vi "Coord window-Offset to zero.vi"() -> (0 "error out":errorcluster)   [LabVIEW 2020]
uses:
  Globals/Coord window-Globals.vi
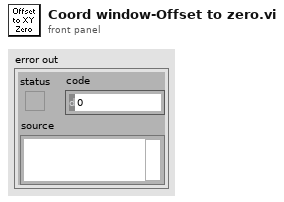
[diagram p1: front panel]
types:
  T1 = typedef "Coordinate list window refs.ctl" = cluster{"Window Name (i.e. Key)":string, "menu reference":refnum<k9>, "VI's reference":refnum<vi>, "Pane 1":refnum<vi>, "Pane 2":refnum<vi>, "Coord Listbox":refnum<vi>, "File name":refnum<vi>, "Picture Map":refnum<vi>, "Stage XYZ Position ind.":refnum<vi>}
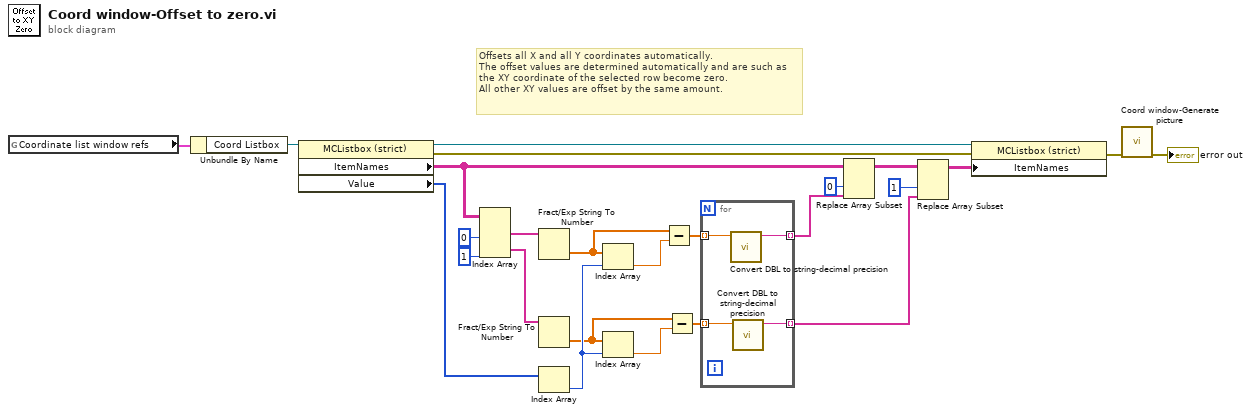
[diagram p0: block diagram]
diagram:
  # "Offsets all X and all Y coordinates automatically.\nThe offset values are determined automatically and are such as the XY coordinate of the selected row become zero.\nAll other XY values are offset by the same amount."
  n1 = global read "Coord window-Globals.vi" "Coordinate list window refs"() -> (w25:T1)
  n2 = Unbundle By Name(w25) -> ("Coord Listbox"=w24:refnum<vi>)
  n3 = property class="MCListbox (strict)"(reference=w24) -> (reference out=w4:refnum<vi>, error out=w3:errorcluster, "ItemNames"=w11:string[][], "Value"=w23:i32[])  [unwired: 1 in]
  n4 = Index Array(array=w11, index (col) #1=0 ("disabled index (col)"), index (col) #2=1 ("index (col)")) -> (element #1=w19:string[], element #2=w18:string[])  [unwired: 2 in]
  n5 = Fract/Exp String To Number(string=w19) -> (number=w17:dbl[])  [unwired: 3 in, 1 out]
  n6 = Fract/Exp String To Number(string=w18) -> (number=w15:dbl[])  [unwired: 3 in, 1 out]
  n7 = Index Array(array=w23) -> (element=w20:i32)  [unwired: 1 in]
  n8 = Index Array(array=w17, index=w20) -> (element=w16:dbl)
  n9 = Index Array(array=w15, index=w20) -> (element=w14:dbl)
  n10 = Subtract(x=w17, y=w16) -> (x-y=w13:dbl[])
  n11 = Subtract(x=w15, y=w14) -> (x-y=w12:dbl[])
  n12 = for {
    tunnel: w13 -> [w29] mode=indexing
    tunnel: w12 -> [w28] mode=indexing
    tunnel: [w27] -> w5 mode=indexing
    tunnel: [w26] -> w8 mode=indexing
    n13 = call <userlib>:"Convert DBL to string-decimal precision.vi"("DBL Value"=w29) -> ("Converted to String"=w27:string)  [unwired: 10 in]
    n14 = call <userlib>:"Convert DBL to string-decimal precision.vi"("DBL Value"=w28) -> ("Converted to String"=w26:string)  [unwired: 10 in]
  }
  n15 = Replace Array Subset(array=w11, new element=w5, index (col)=0 ("disabled index (col)")) -> (w9:string[][])  [unwired: 1 in]
  n16 = Replace Array Subset(array=w9, new element=w8, index (col)=1 ("disabled index (col)")) -> (w6:string[][])  [unwired: 1 in]
  n17 = property class="MCListbox (strict)"(reference=w4, error in=w3, "ItemNames"=w6) -> (error out=w2:errorcluster)  [unwired: 1 out]
  n18 = call "Coord window-Generate picture.vi"("error in (no error)"=w2) -> ("error out"=→"error out":errorcluster)  [unwired: 10 in]
